vi "Calculate Spectrum.vi"(0 "input data":cdb[](array[numeric]), 1 "window parameter":dbl=nan, 2 "window":T1=1 items=["Rectangle"=0, "Hanning"=1, "Hamming"=2, "Blackman-Harris"=3, "Exact Blackman"=4, "Blackman"=5, "Flat Top"=6, "4 Term B-Harris "=7, "7 Term B-Harris"=8, "Low Sidelobe"=9, "Blackman Nuttall"=11, "Triangle"=30, "Bartlett-Hanning"=31, "Bohman"=32, "Parzen"=33, "Welch"=34, "Kaiser"=60, "Dolph-Chebyshev"=61, "Gaussian"=62], 11 "error in":errorcluster, 13 "IQ rate":dbl=1.0 format="%#_6p") -> (4 "spectrum output":cluster{"Ramp Pattern":dbl[], dbl[]}(graph), 15 "error out":errorcluster)   [LabVIEW 2019]
uses:
  <vilib>/Analysis/4window.llb/windowTd.ctl
  <vilib>/Analysis/1siggen.llb/Ramp Pattern by Samples.vi
  <vilib>/Analysis/2dsp.llb/Complex FFT.vi
  <vilib>/Analysis/0measdsp.llb/Scaled Time Domain Window (CDB).vi
  <vilib>/Analysis/NI_AALPro.lvlib
  <vilib>/Analysis/NI_AALBase.lvlib
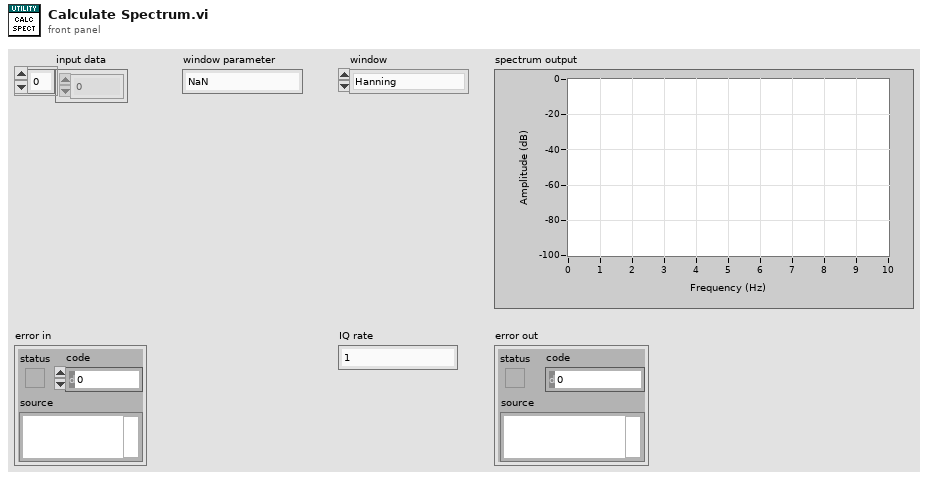
[diagram p1: front panel]
types:
  T1 = typedef "NI_AALPro.lvlib/windowTd.ctl" = u32
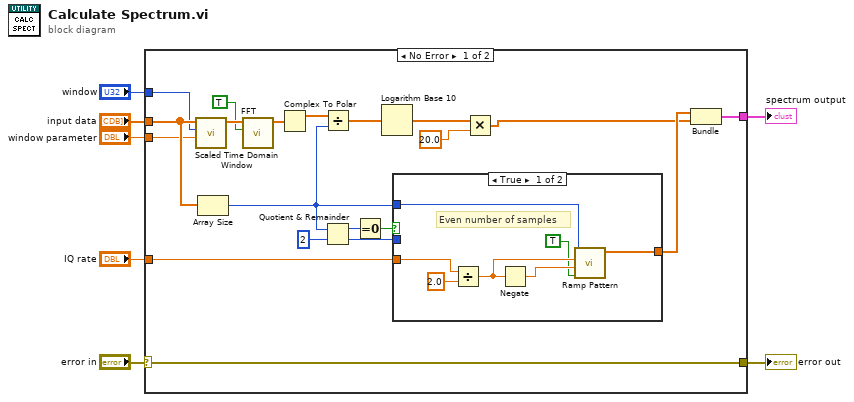
[diagram p0: block diagram]
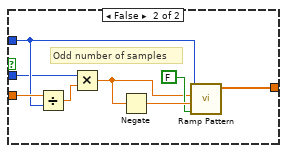
[diagram p2: hidden frame]
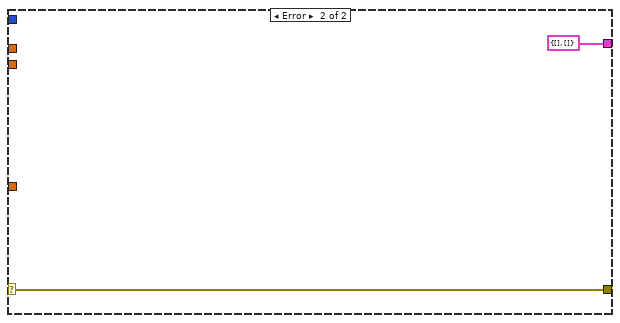
[diagram p3: hidden frame]
diagram:
  n1 = case shown="No Error" "error in" {
    selector: "error in" -> [w23 w44]
    tunnel: [w23 w44] -> w6
    tunnel: [w16 cluster{"Ramp Pattern":dbl[], dbl[]} {"Ramp Pattern"=[], []}] -> w1
    tunnel: "input data" -> [w15 _]
    tunnel: "window parameter" -> [w14 _]
    tunnel: "window" -> [w13 _]
    tunnel: "IQ rate" -> [w12 _]
    frame No Error {
      n2 = call-poly <vilib>:"Scaled Time Domain Window.vi"("window parameter"=w14, "window"=w13, "X"=w15) -> ("Windowed X"=w27:cdb[])  [unwired: 6 in, 2 out]
      n3 = Array Size(array=w15) -> (size(s)=w18:i32)
      n4 = call-poly <vilib>:"FFT.vi"("shift?"=TRUE, "X"=w27) -> ("FFT {X}"=w25:cdb[])  [unwired: 8 in, 1 out]
      n5 = Complex To Polar(r * e^(i*theta)=w25) -> (r=w24:dbl[])  [unwired: 1 out]
      n6 = Divide(x=w24, y=w18) -> (x/y=w11:dbl[])
      n7 = Quotient & Remainder(x=w18, y=2) -> (x-y*floor(x/y)=w20:i32, floor(x/y)=w22:i32)
      n8 = Equal To 0?(x=w20) -> (x = 0?=w21:bool)
      n9 = Logarithm Base 10(1:w11) -> (0:w10:dbl[])
      n10 = case shown="True" w21 {
        tunnel: w18 -> [w30 w38]
        tunnel: [w29 w40] -> w17
        tunnel: w12 -> [w28 w39]
        tunnel: w22 -> [_ w37]
        frame True {
          # "Even number of samples"
          n11 = Divide(x=w28, y=2.0) -> (x/y=w32:dbl)
          n12 = Negate(x=w32) -> (-x=w33:dbl)
          n13 = call-poly <vilib>:"Ramp Pattern.vi"("exclude end?"=TRUE, "start"=w33, "end"=w32, "samples"=w30) -> ("Ramp Pattern"=w29:dbl[])  [unwired: 6 in, 1 out]
        }
        frame False {
          # "Odd number of samples"
          n14 = Divide(x=w39, y=w38) -> (x/y=w36:dbl)
          n15 = Multiply(x=w37, y=w36) -> (x*y=w35:dbl)
          n16 = Negate(x=w35) -> (-x=w42:dbl)
          n17 = call-poly <vilib>:"Ramp Pattern.vi"("exclude end?"=FALSE, "start"=w42, "end"=w35, "samples"=w38) -> ("Ramp Pattern"=w40:dbl[])  [unwired: 6 in, 1 out]
        }
      }
      n18 = Multiply(x=w10, y=20.0) -> (x*y=w8:dbl[])
      n19 = Bundle("Ramp Pattern"=w17, w8) -> (w16:cluster{"Ramp Pattern":dbl[], dbl[]})  [unwired: 1 in]
    }
    frame Error {
    }
  }
  "error out" <- w6
  "spectrum output" <- w1
